vi "finishKeeperPassToStriker.vi"(9 "Game":refnum<class "Game.lvclass">, 10 "OffesiveTeam":refnum<class "Ally.lvclass">, 11 "KeeperPassToStrikerPlay in":refnum<class "KeeperPassToStrikerPlay.lvclass">) -> (2 "finishKeeperPassToStriker":bool, 3 "KeeperPassToStrikerPlay out":refnum<class "KeeperPassToStrikerPlay.lvclass">)   [LabVIEW 2024, in "KeeperPassToStrikerPlay.lvclass"]
uses:
  KeeperPassToStrikerPlay.lvclass
  Ally_class/Ally.lvclass
  C:/Users/ROBOIME2/Documents/SSL ROBOIME/SSL_AI/Team_class/Team.lvclass
  Game_class/Game.lvclass
  Referee_class/command_interpreted.ctl
  Robot_class/roles.ctl
  Utilities_class/Utilities.lvclass
  Team_class/Team.lvclass/Team.ctl
  Game_class/Game.lvclass/Game.ctl
  Referee_class/Referee.lvclass/Referee.ctl
  Object_class/Object.lvclass/Object.ctl
  Events_class/Events.lvclass/Events.ctl
  Game_class/Read EventsRef.vi
  Game_class/Read Referee.vi
  Referee_class/Read our_goalie_id.vi
  Events_class/Read touch.vi
  Events_class/Read id_touch.vi
  Game_class/Read BallRef.vi
  Object_class/Read x.vi
  Referee_class/Read command_interpreted.vi
  Team_class/Read RobotRef.vi
  Team_class/Read OffensivePlay Finished.vi
  Ball_class/Ball.lvclass
  C:/Users/ROBOIME2/Documents/SSL ROBOIME/SSL_AI/Object_class/Object.lvclass
  Robot_class/Robot.lvclass
  Referee_class/Referee.lvclass
  Events_class/Events.lvclass
panel:
  out "error out":errorcluster
  in  "error in (no error)":errorcluster
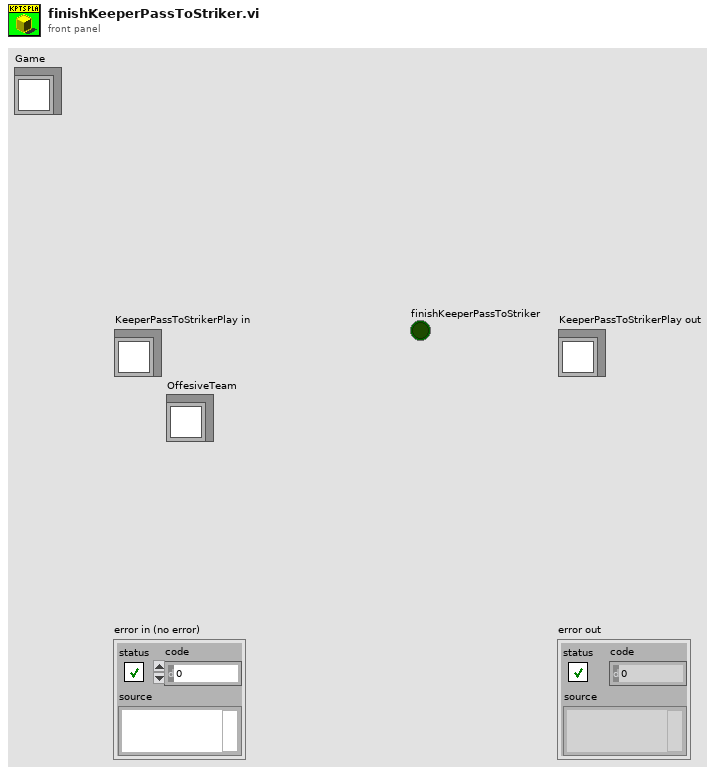
[diagram p1: front panel]
types:
  T1 = typedef "roles.ctl" = enum16{"SimpleBallPlacement", "BallPlacementAllyPasser", "BallPlacementAllyReceiver", "BallPlacementEnemy", "5Robots5th", "PassBestReceiver", "5Robots4th", "5Robots3rd", "5Robots2nd", "5Robots1st", "PassBestRobot", "WaitPass", "ABCThirdKicker", "ABCFirstKicker", "ABCSecondKicker", "Tabler", "TableFinalizer", "PrepareRollToPassRoller", "PrepareRollToPassReceiver", "SimplePassRoll", "SimplePassRollReceiver", "PenaltyDefense", "PreparePassReceiver 2", "PreparePassReceiver 1", "PassObserver", "Timeout", "Goto", "ZigZag", "None", "BallOutOfField", "DefenderArea", "Duelist", "AttackerStop", "FollowAttacker", "KeeperRole", "KickPenalty", "AttackerAimGoal", "AttackerBlock", "Marker", "Halt", "Shoot", "PassKicker", "PassReceiver", "TestRole", "PenaltyAttacker"}
  T2 = typedef "command_interpreted.ctl" = enum16{"Goal Ally", "Goal Enemy", "Ball Placement Enemy", "Ball Placement Ally", "Normal Half Time", "Extra Time  Break", "Extra Half Time", "None", "Post Game", "PKA Normal Start", "Prepare Kickoff Ally", "PKE Normal Start", "Prepare Kickoff Enemy", "Force Start", "Halt", "Timeout", "Prepare Penalty Ally", "Prepare Penalty Enemy", "PPA NormalStart", "PPE Normal Start", "Indirect Free Ally", "Direct Free Enemy", "Direct Free Ally", "Indirect Free Enemy", "Stop"}
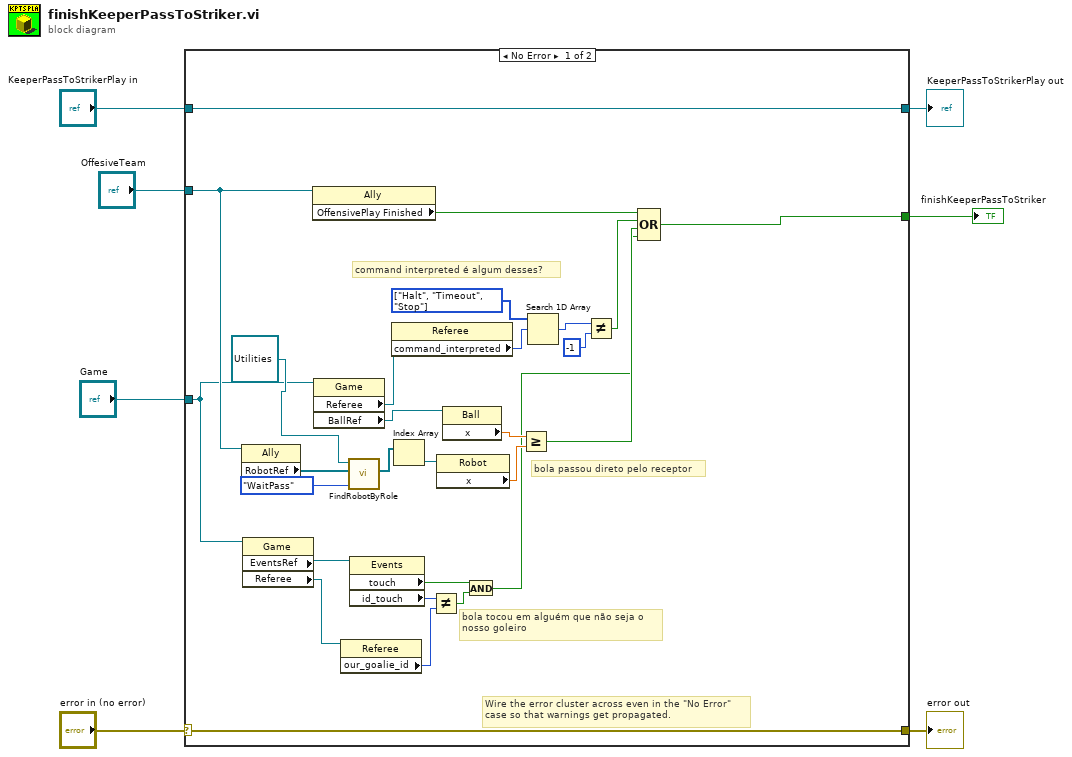
[diagram p0: block diagram]
diagram:
  n1 = case shown="No Error" "error in (no error)" {
    selector: "error in (no error)" -> [w34 w37]
    tunnel: [w34 w37] -> w6
    tunnel: [w35 w36] -> w4
    tunnel: "KeeperPassToStrikerPlay in" -> [w35 w36]
    tunnel: "OffesiveTeam" -> [w21 _]
    tunnel: [w32 _] -> w2
    tunnel: "Game" -> [w17 _]
    frame No Error {
      w30 = T2[] [enum."Halt", enum."Timeout", enum."Stop"] items=["Goal Ally", "Goal Enemy", "Ball Placement Enemy", "Ball Placement Ally", "Normal Half Time", "Extra Time  Break", "Extra Half Time", "None", "Post Game", "PKA Normal Start", "Prepare Kickoff Ally", "PKE Normal Start", "Prepare Kickoff Enemy", "Force Start", "Halt", "Timeout", "Prepare Penalty Ally", "Prepare Penalty Enemy", "PPA NormalStart", "PPE Normal Start", "Indirect Free Ally", "Direct Free Enemy", "Direct Free Ally", "Indirect Free Enemy", "Stop"] ("Array")
      # "command interpreted é algum desses?"
      # "bola tocou em alguém que não seja o\nnosso goleiro"
      # "bola passou direto pelo receptor"
      # "Wire the error cluster across even in the \"No Error\"\ncase so that warnings get propagated."
      n2 = property class="Ally"(reference=w21) -> ("RobotRef"=w20:refnum<class "Robot.lvclass">[])  [unwired: 1 in, 2 out]
      n3 = property class="Game"(reference=w17) -> ("EventsRef"=w16:refnum<class "Events.lvclass">, "Referee"=w11:refnum<class "Referee.lvclass">)  [unwired: 1 in, 2 out]
      n4 = property class="Ally"(reference=w21) -> ("OffensivePlay Finished"=w33:bool)  [unwired: 1 in, 2 out]
      n5 = property class="Game"(reference=w17) -> ("Referee"=w9:refnum<class "Referee.lvclass">, "BallRef"=w27:refnum<class "Ball.lvclass">)  [unwired: 1 in, 2 out]
      n6 = property class="Referee"(reference=w11) -> ("our_goalie_id"=w10:i32)  [unwired: 1 in, 2 out]
      n7 = call "FindRobotByRole.vi"("role"=roles."WaitPass", "RobotRef"=w20, "Utilities in"=refnum<class "Utilities.lvclass"> refnum) -> ("Robots"=w25:refnum<class "Robot.lvclass">[])  [unwired: 5 in, 3 out]
      n8 = property class="Events"(reference=w16) -> ("touch"=w15:bool, "id_touch"=w12:i32)  [unwired: 1 in, 2 out]
      n9 = property class="Referee"(reference=w9) -> ("command_interpreted"=w8:T2)  [unwired: 1 in, 2 out]
      n10 = Index Array(array=w25) -> (element=w24:refnum<class "Robot.lvclass">)  [unwired: 1 in]
      n11 = Not Equal?(x=w12, y=w10) -> (x != y?=w13:bool)
      n12 = property class="Robot"(reference=w24) -> ("x"=w23:dbl)  [unwired: 1 in, 2 out]
      n13 = property class="Ball"(reference=w27) -> ("x"=w26:dbl)  [unwired: 1 in, 2 out]
      n14 = And(x=w15, y=w13) -> (x .and. y?=w14:bool)
      n15 = Greater Or Equal?(x=w26, y=w23) -> (x >= y?=w22:bool)
      n16 = Search 1D Array(1D array=w30, element=w8) -> (index of element=w31:i32)  [unwired: 1 in]
      n17 = Not Equal?(x=w31, y=-1) -> (x != y?=w28:bool)
      n18 = Compound Arithmetic op=OR(w33, w28, w22, w14) -> (w32:bool)
    }
    frame Error {
    }
  }
  "error out" <- w6
  "KeeperPassToStrikerPlay out" <- w4
  "finishKeeperPassToStriker" <- w2
